vi "QueryServer_Query_SetResponse.vi"(0 "gRPCid":T2, 1 "message":string, 2 "status":i32, 3 "error in (no error)":errorcluster) -> (10 "error out":errorcluster)   [LabVIEW 2019]
uses:
  QueryServer_gRPCid.ctl
  QueryServer_QueryResponse.ctl
  Debug/labview_query_server.dll
panel:
  in  "QueryResponse":T1
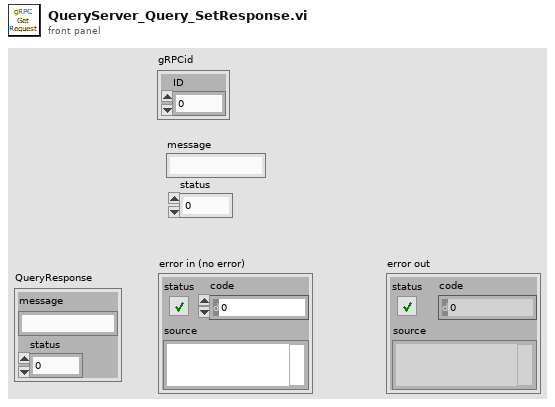
[diagram p1: front panel]
types:
  T1 = typedef "QueryServer_QueryResponse.ctl" = cluster{"message":string, "status":i32}
  T2 = typedef "QueryServer_gRPCid.ctl" = cluster{"ID":u64}
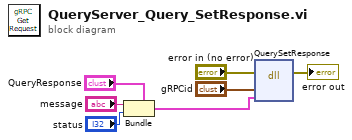
[diagram p0: block diagram]
diagram:
  n1 = Bundle(cluster="QueryResponse", "message"="message", "status"="status") -> (w3:T1)
  n2 = dll-call lib="C:/dev/labview-grpc-query-server/Debug/labview_query_server.dll" fn="QuerySetResponse"(error in="error in (no error)", "id"="gRPCid", "data"=w3) -> (error out=→"error out":errorcluster)  [unwired: 5 in, 1 out]
